vi "TestForScaleInImageTextbox.vi"() -> ()   [LabVIEW 2013]
uses:
  Mag.ctl
  TextOnImage.ctl
  <vilib>/vision/NI_Vision_Development_Module.lvlib
panel:
  in  "File Path":path
  in  "Mag":T1
  in  "High Resolution":bool
  out "Image":T2(plugin-control)
  out "Status of Temperature Controller":string="Setpoint"
  in  "Setpoint (°C)":dbl=28.0 min=-50.0 max=50.0 step=0.1 format="%.1g °C"
  out "Temp String (C)":string="27.0"
  out "Experiment Name":string
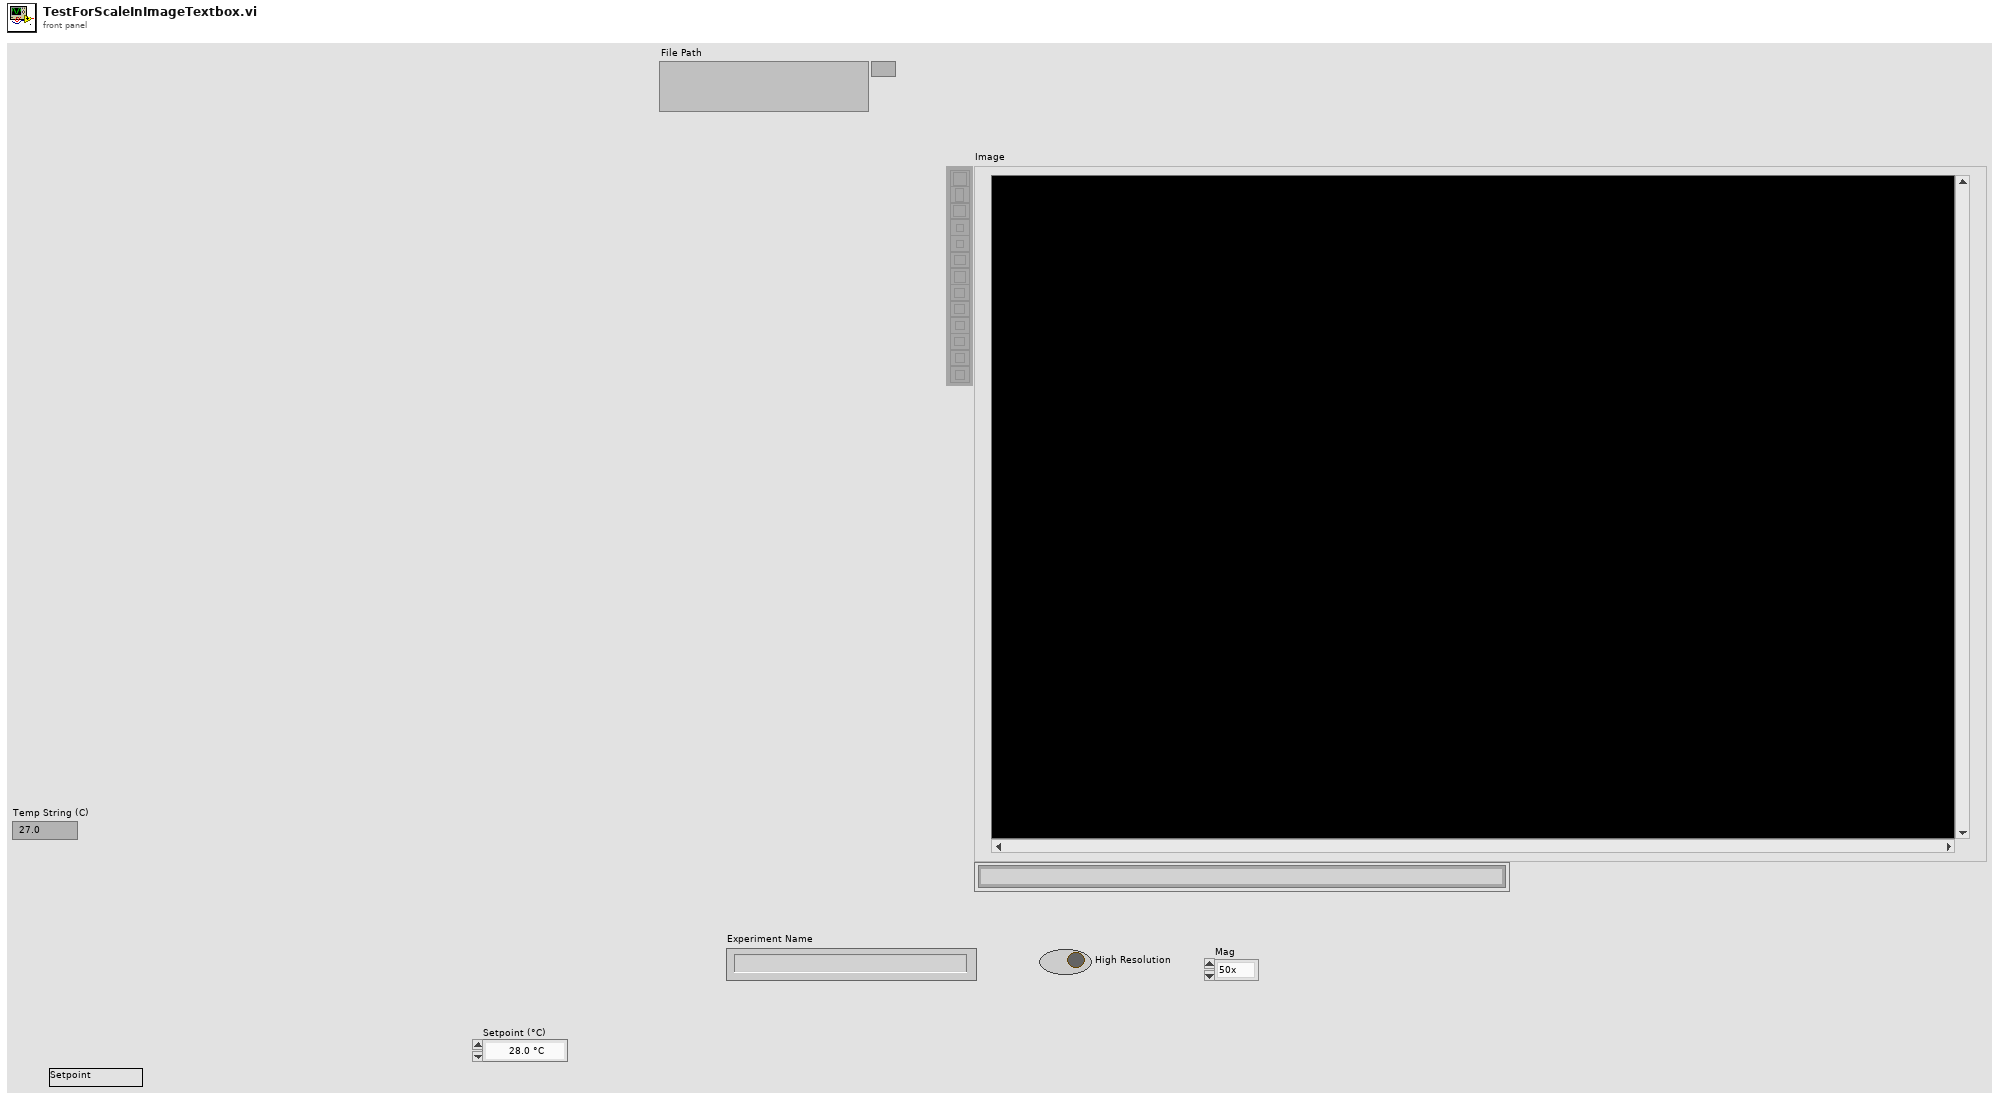
[diagram p1: front panel]
types:
  T1 = typedef "Mag.ctl" = enum16{"50x", "20x_S", "20x", "4x"}
  T2 = typedef "IMAQ Image.ctl" = refnum<image>
  T3 = typedef "TextOnImage.ctl" = cluster{"Status":string, "Experiment Name":string, "Current Temp (C)":string, "Mag":string, "Set Point (C)":string, "Cooling Rate (C/min)":string}
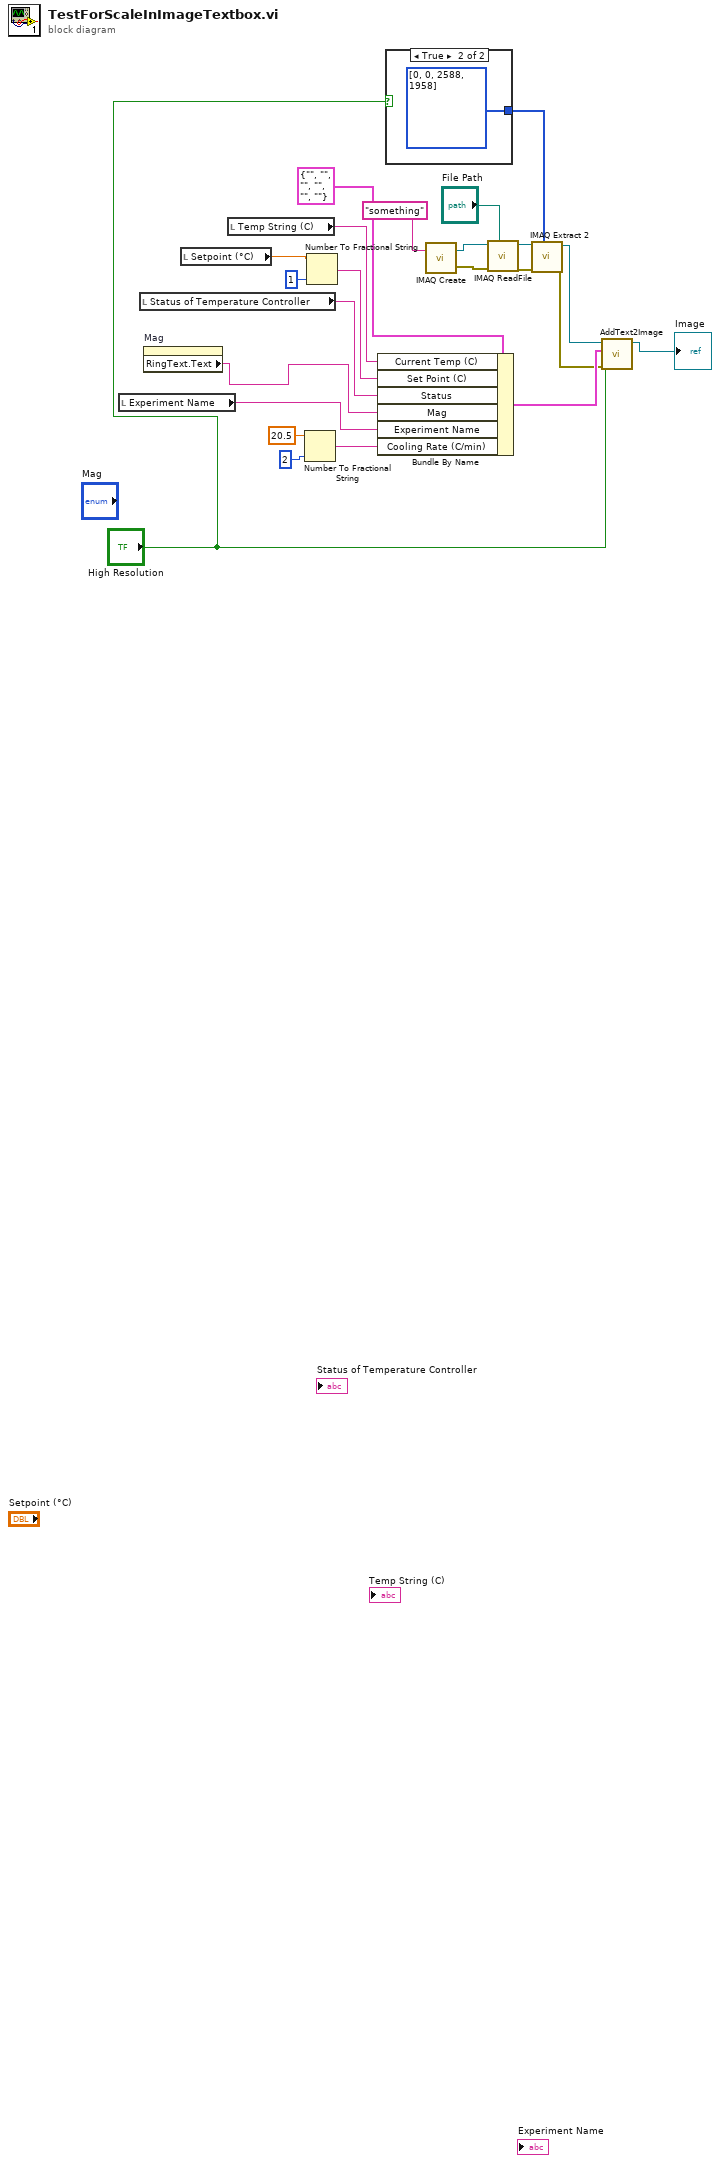
[diagram p0: block diagram]
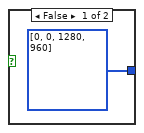
[diagram p2: hidden frame]
diagram:
  n1 = local read "Experiment Name"() -> (w20:string)
  n2 = local read "Status of Temperature Controller"() -> (w16:string)
  n3 = property on="Mag" class="Enum (strict)"() -> ("RingText.Text"=w8:string)  [unwired: 2 in, 2 out]
  n4 = local read "Setpoint (°C)"() -> (w21:dbl)
  n5 = local read "Temp String (C)"() -> (w17:string)
  n6 = Number To Fractional String(number=20.5, precision (6)=i16 2) -> (F-format string=w19:string)  [unwired: 2 in]
  n7 = Number To Fractional String(number=w21, precision (6)=i16 1) -> (F-format string=w22:string)  [unwired: 2 in]
  n8 = Bundle By Name(cluster=T3 {"Status"="", "Experiment Name"="", "Current Temp (C)"="", "Mag"="", "Set Point (C)"="", "Cooling Rate (C/min)"=""} ("TextOnImage"), "Current Temp (C)"=w17, "Set Point (C)"=w22, "Status"=w16, "Mag"=w8, "Experiment Name"=w20, "Cooling Rate (C/min)"=w19) -> (w14:T3)
  n9 = case shown="True" "High Resolution" {
    tunnel: [i32[] [0, 0, 1280, 960] ("Optional Rectangle") i32[] [0, 0, 2588, 1958] ("Optional Rectangle")] -> w2
    frame False {
    }
    frame True {
    }
  }
  n10 = call "IMAQ Create"("Image Name"="something") -> ("New Image"=w11:T2, "error out"=w13:errorcluster)  [unwired: 4 in]
  n11 = call "IMAQ ReadFile"("File Path"="File Path", "error in (no error)"=w13, "Image"=w11) -> ("error out"=w4:errorcluster, "Image Out"=w6:T2)  [unwired: 4 in, 3 out]
  n12 = call "IMAQ Extract 2"("Optional Rectangle"=w2, "error in (no error)"=w4, "Image Src"=w6) -> ("error out"=w3:errorcluster, "Image Dst Out"=w5:T2)  [unwired: 7 in]
  n13 = call "AddText2Image.vi"("error in (no error)"=w3, "High Resolution"="High Resolution", "TextOnImage"=w14, "Input Image"=w5) -> ("Output Image"=→"Image":T2)  [unwired: 6 in, 1 out]
